vi "Narrowband Filter Design and Processing.vi"() -> ()   [LabVIEW 2023]
doc: "Demonstrates how to use the DFD Narrowband Filter Design VI, the DFD Plot Narrowband Freq Response VI, and the DFD Narrowband Filtering VI to design, analyze, and implement a narrowband filter.\n\nComplete the following steps to use this VI.\n1) Run the VI.\n2) Change the specifications.\n3) Observe the Filter Magnitude Response graph to view the overall magnitude response.\n4) Change the <B>Signal Frequency</B> value.\n5) Observe the waveforms of the original and filtered signals on the Signals graph. If you set the signal frequency within the passband, the two waveforms are nearly identical except for a delay. If you set the signal frequency within the stopband, the filtered signal is attenuated significantly.\n6) Observe the <B>Attenuation</B> output to view the actual attenuation of the filtered signal compared to the original one.\n7) Click the <B>STOP</B> button to stop this VI."
uses:
  <vilib>/addons/Digital Filter Design/_Objects.llb/DFD Filter Frequence Specification (Design).ctl
  <vilib>/addons/Digital Filter Design/_Objects.llb/DFD Filter Ripple Specification (Design).ctl
  <vilib>/Analysis/5stat.llb/RMS (DBL).vi
  <vilib>/addons/Digital Filter Design/Multirate.llb/DFD Narrowband Filtering (Array).vi
  <vilib>/Analysis/NI_AALBase.lvlib
  <vilib>/addons/Digital Filter Design/NI_DigFilterLicensed.lvlib
  <vilib>/Analysis/NI_AALPro.lvlib
panel:
  out "Attenuation [dB]":dbl format="%.2g"
  in  "stop":bool
  out "Error Message":string
  out "Signals":dbl[][](graph)
  out "Magnitude Response":cluster{"f0":dbl, "df":dbl, "magnitude":dbl[]}(graph)
  in  "Signal Frequency [Hz]":dbl=0.004
  in  "Filter Type":u16(ring) items=["Lowpass", "Highpass", "Bandpass", "Bandstop"]
  in  "Sampling Frequency [Hz]":dbl=1.0 format="%.2f"
  in  "Ripple Specifications":T1={"passband"=0.1, "stopband"=60.0, "dB/linear? (T: dB)"=TRUE}
  in  "Frequency Specifications [Hz]":T2={"fpass 1"=0.015, "fstop 1"=0.02, "fpass 2 "=0.0, "fstop 2"=0.0}
  # "Select Help>>Show Context Help and move the cursor over the VI icon for more information."
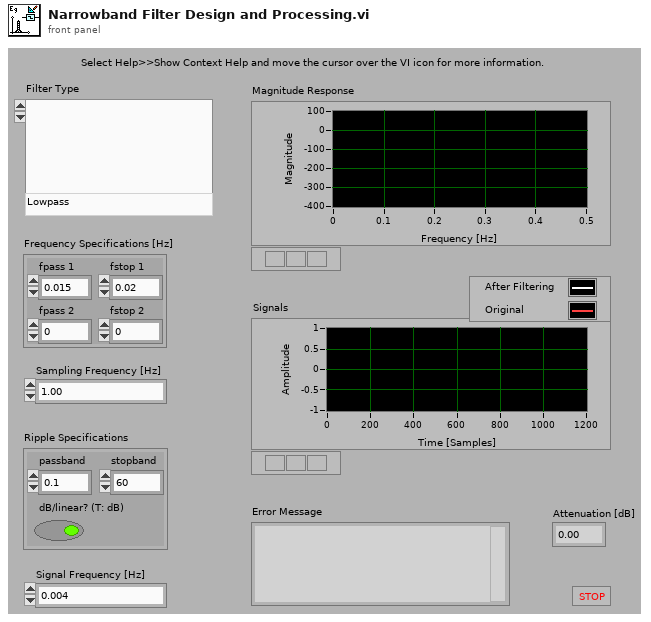
[diagram p1: front panel]
types:
  T1 = typedef "NI_DigFilterLicensed.lvlib/DFD Filter Ripple Specification (Design).ctl" = cluster{"passband":dbl, "stopband":dbl, "dB/linear? (T: dB)":bool}
  T2 = typedef "NI_DigFilterLicensed.lvlib/DFD Filter Frequence Specification (Design).ctl" = cluster{"fpass 1":dbl, "fstop 1":dbl, "fpass 2 ":dbl, "fstop 2":dbl}
  T3 = typedef "NI_DigFilterLicensed.lvlib/DFD Narrowband Filter Obj.ctl" = cluster{"multirate filters":T4[], "filter type":enum32{"Lowpass", "Highpass", "Bandpass", "Bandstop", "Wideband-Lowpass", "Wideband-Highpass"}}
  T4 = typedef "NI_DigFilterLicensed.lvlib/DFD Multirate Filter Obj.ctl" = cluster{"mMRate_Structure":enum16{"CIC", "FIR", "IIR", "Lattice"}, "mMRate_Mode":T5, "mMRate_Factor":i32, "mMRate_FIRParams":cluster{"mMRate_FIR_H":dbl[], "mMRate_FIR_IsNyquist?":bool, "mMRate_FIR_IsSymmetric?":bool}, "mMRate_CICParams":cluster{"mMRate_CIC_#Stage":i32, "mMRate_CIC_Lag":i32, "mMRate_CIC_Type":enum16{"Lowpass", "Highpass"}}, "mMRate_Order":i32, "mMRate_Version":string, "mMRate_Comments":string, "mMRate_RationalFactor":cluster{"mMRate_L":i32, "mMRate_M":i32}, "mMRate_Fs":dbl, "mMRate_Quantized?":bool, "mMRate_QFilterGain":dbl, "mMRate_CoefWl":i16, "mMRate_Scaling":cluster{"mMRate_ScaleByPowerOf2?":bool, "mMRate_ScaleType":T6}, "mMRate_InputWl":i16, "mMRate_OutputWl":i16, "mMRate_OutputMode":T7, "mMRate_MultMode":T8, "mMRate_BitPruning":bool, "mMRate_GainWl":i16, "mMRate_OutputFwl":i16, "mMRate_SumIwl":i16, "mMRate_InputIwl ":i16, "mMRate_SumWl":i16, "mMRate_CoefIwl":i16}
  T5 = typedef "NI_DigFilterLicensed.lvlib/DFD Multirate Mode.ctl" = i16
  T6 = typedef "NI_DigFilterLicensed.lvlib/DFD Coef Norm Type.ctl" = enum16{"No Norm", "Time Domain 1-Norm", "Time Domain 2-Norm", "Time Domain Inf-Norm"}
  T7 = typedef "NI_DigFilterLicensed.lvlib/DFD Round-off Mode.ctl" = enum16{"Nearest", "Truncation"}
  T8 = typedef "NI_DigFilterLicensed.lvlib/DFD FXP MRate Multiply Mode.ctl" = enum16{"Truncated", "Full"}
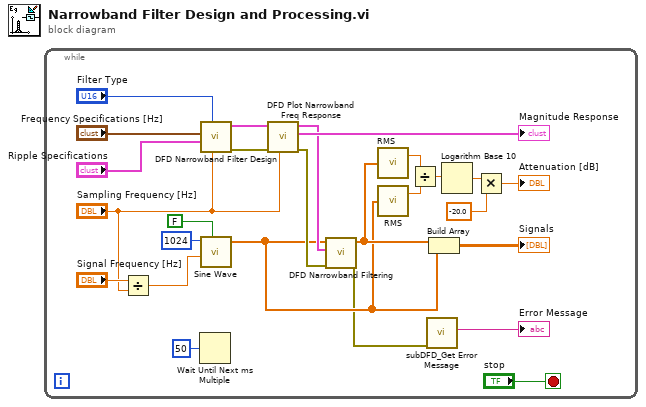
[diagram p0: block diagram]
diagram:
  n1 = while {
    stop <- "stop" stop-if-true
    n2 = Divide(x="Signal Frequency [Hz]", y="Sampling Frequency [Hz]") -> (x/y=w12:dbl)
    n3 = Wait Until Next ms Multiple(millisecond multiple=u32 50) -> ()  [unwired: 1 out]
    n4 = call <vilib>:"DFD Narrowband Filter Design.vi"("fs [Hz]"="Sampling Frequency [Hz]", "filter type"="Filter Type", "ripple specs"="Ripple Specifications", "freq specs [Hz]"="Frequency Specifications [Hz]") -> ("error out"=w23:errorcluster, "narrowband filter out"=w24:T3)  [unwired: 1 in, 5 out]
    n5 = call <vilib>:"Sine Wave.vi"("samples"=1024, "frequency"=w12, "reset phase"=FALSE) -> ("sine wave"=w10:dbl[])  [unwired: 2 in, 2 out]
    n6 = call <vilib>:"DFD Plot Narrowband Freq Response.vi"("fs [Hz]"="Sampling Frequency [Hz]", "error in (no error)"=w23, "narrowband filter in"=w24) -> ("error out"=w19:errorcluster, "magnitude response"=→"Magnitude Response":cluster{"f0":dbl, "df":dbl, "magnitude":dbl[]}, "narrowband filter out"=w20:T3)  [unwired: 3 in, 3 out]
    n7 = call-poly <vilib>:"DFD Narrowband Filtering.vi"("error in (no error)"=w19, "narrowband filter"=w20, "signal in"=w10) -> ("error out"=w2:errorcluster, "signal out"=w11:dbl[])  [unwired: 1 in, 6 out]
    n8 = call-poly <vilib>:"RMS.vi"("X"=w11) -> ("rms value"=w8:dbl)  [unwired: 1 out]
    n9 = call-poly <vilib>:"RMS.vi"("X"=w10) -> ("rms value"=w9:dbl)  [unwired: 1 out]
    n10 = Divide(x=w8, y=w9) -> (x/y=w7:dbl)
    n11 = call <vilib>:"subDFD_Get Error Message.vi"("error in (no error)"=w2) -> ("Error Message"=→"Error Message":string)  [unwired: 10 out]
    n12 = Build Array(w11, w10) -> (→"Signals":dbl[][])
    n13 = Logarithm Base 10(1:w7) -> (0:w6:dbl)
    n14 = Multiply(x=w6, y=-20.0) -> (x*y=→"Attenuation [dB]":dbl)
  }
